vi "MessageName.vi"() -> (2 "MessageName":string)   [LabVIEW 2020, in "CmdDigitalMultiple.lvlib"]
uses:
  CmdDigitalMultiple.lvlib
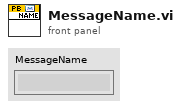
[diagram p1: front panel]
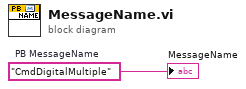
[diagram p0: block diagram]
diagram:
  w1 = "CmdDigitalMultiple"  # PB MessageName
  "MessageName" <- w1
